vi "Parse Notes.vi"(8 "error in":errorcluster, 11 "string in":string) -> (0 "error out":errorcluster, 1 "Done Reading?":bool, 2 "sr note out":string[](array[string]), 3 "result string out":string)   [LabVIEW 2018]
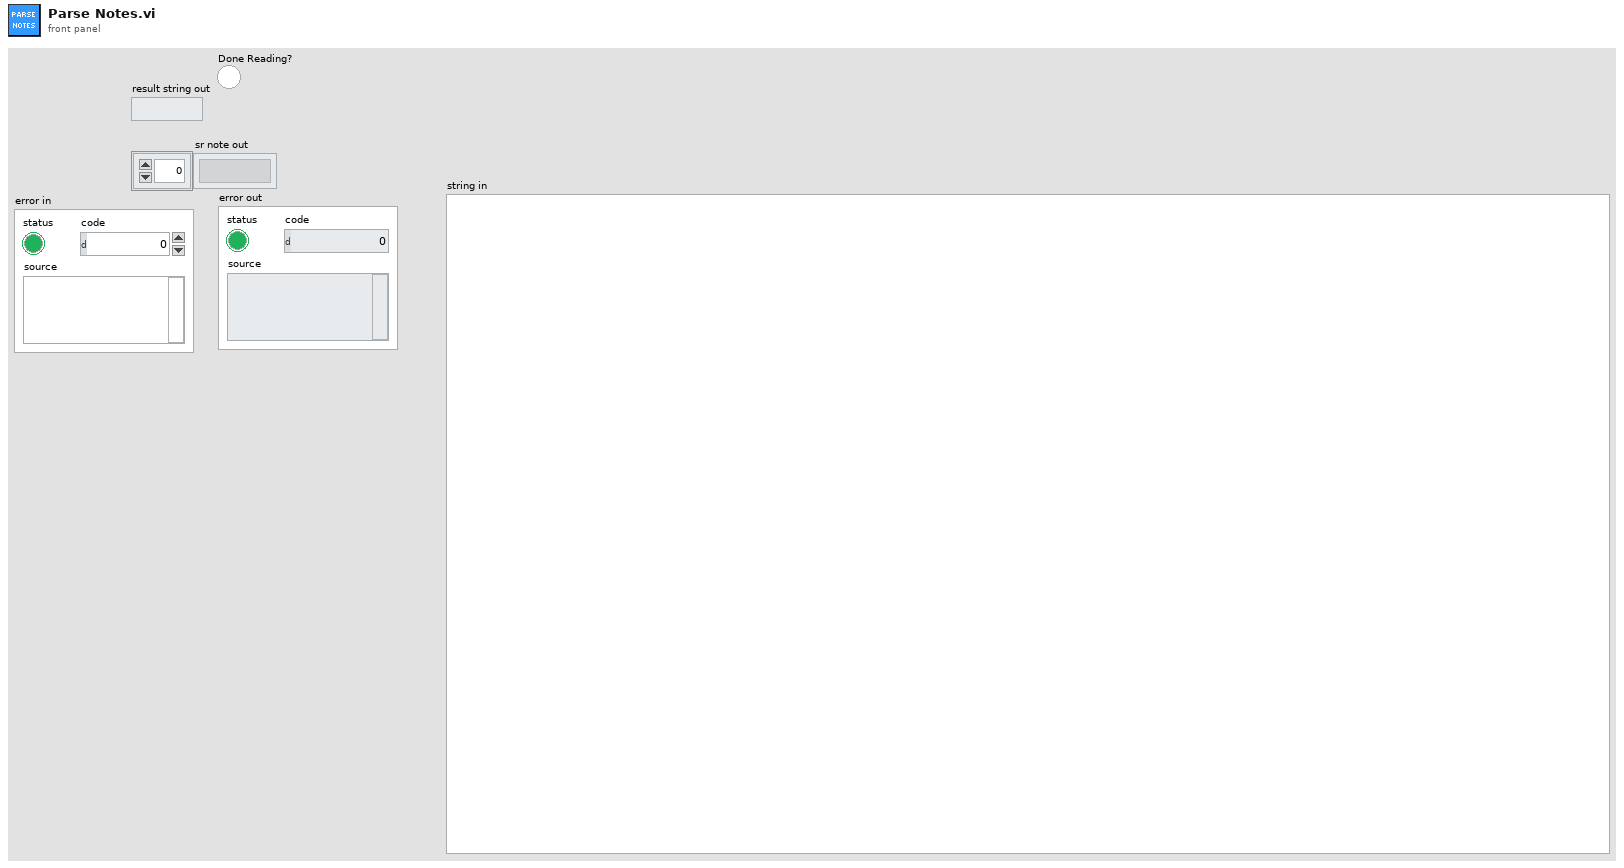
[diagram p1: front panel]
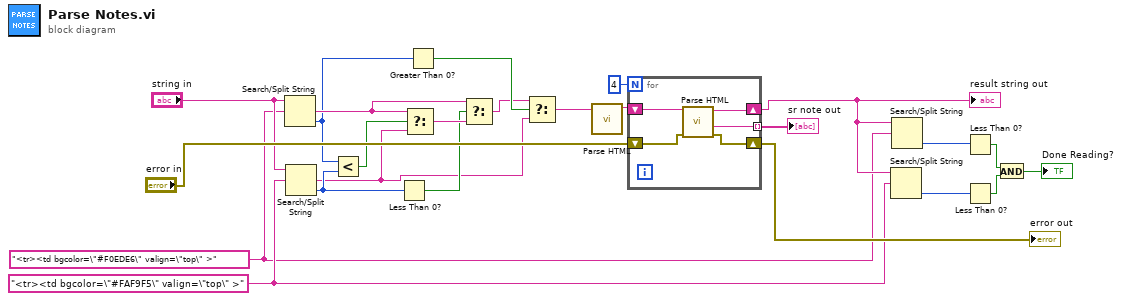
[diagram p0: block diagram]
diagram:
  w13 = "<tr><td bgcolor=\"#FAF9F5\" valign=\"top\" >" ("search string/char (-)")
  w11 = "<tr><td bgcolor=\"#F0EDE6\" valign=\"top\" >" ("search string/char (-)")
  n1 = Search/Split String(string="string in", search string/char (-)=w11) -> (match + rest of string=w8:string, offset of match=w5:i32)  [unwired: 1 in, 1 out]
  n2 = Search/Split String(string="string in", search string/char (-)=w13) -> (match + rest of string=w2:string, offset of match=w7:i32)  [unwired: 1 in, 1 out]
  n3 = Less?(x=w5, y=w7) -> (x < y?=w18:bool)
  n4 = Less Than 0?(x=w7) -> (x < 0?=w6:bool)
  n5 = Select(t=w8, s=w18, f=w2) -> (s? t:f=w9:string)
  n6 = Greater Than 0?(x=w5) -> (x > 0?=w4:bool)
  n7 = Select(t=w8, s=w6, f=w9) -> (s? t:f=w3:string)
  n8 = Select(t=w3, s=w4, f=w2) -> (s? t:f=w1:string)
  n9 = call "Parse HTML.vi"("result string in"=w1) -> ("result string out"=w22:string)  [unwired: 8 in, 2 out]
  n10 = for {
    N: 4 -> [_]
    shift-right: [w28] -> w12
    shift-left: w22 -> [w29]
    tunnel: [w27] -> w24 mode=indexing
    shift-right: [w25] -> w19
    shift-left: "error in" -> [w26]
    n11 = call "Parse HTML.vi"("error in"=w26, "result string in"=w29) -> ("error out"=w25:errorcluster, "data"=w27:string, "result string out"=w28:string)  [unwired: 7 in]
  }
  "result string out" <- w12
  "sr note out" <- w24
  "error out" <- w19
  n12 = Search/Split String(string=w12, search string/char (-)=w13) -> (offset of match=w10:i32)  [unwired: 1 in, 2 out]
  n13 = Search/Split String(string=w12, search string/char (-)=w11) -> (offset of match=w21:i32)  [unwired: 1 in, 2 out]
  n14 = Less Than 0?(x=w21) -> (x < 0?=w15:bool)
  n15 = Less Than 0?(x=w10) -> (x < 0?=w16:bool)
  n16 = And(x=w15, y=w16) -> (x .and. y?=→"Done Reading?":bool)
